vi "isolateNextStringElement.vi"(6 "Final Delimiter":T1, 8 "error in (no error)":errorcluster, 10 "inputString":string, 11 "ILC in":refnum<class "ILC.lvclass">) -> (0 "error out":errorcluster, 1 "remainingString":string, 2 "extractedSegment":string, 3 "ILC out":refnum<class "ILC.lvclass">)   [LabVIEW 2013, in "ILCCommon.lvlib" / "ILC.lvclass"]
uses:
  <userlib>/Common/ILC/ILC/ILC.lvclass
  <userlib>/Common/ILC/ILCModelTypedefs/FinalDelimiter.ctl
  <userlib>/Common/ILC/ILCModelTypedefs/ILCModelTypedefs.lvlib
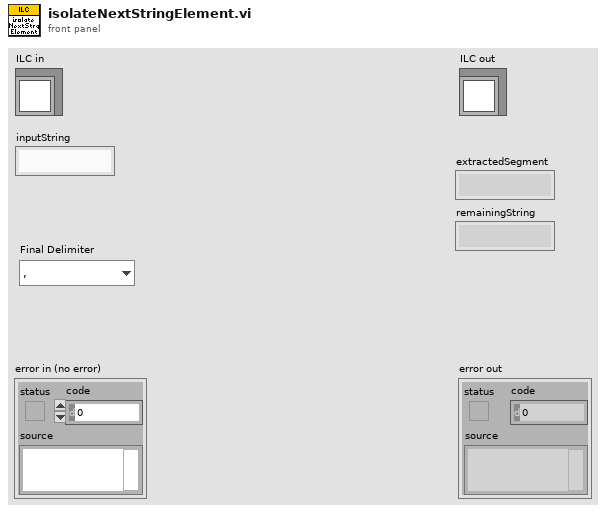
[diagram p1: front panel]
types:
  T1 = typedef "ILCCommon.lvlib/ILCModelTypedefs.lvlib/FinalDelimiter.ctl" = enum16{",", "<CR><LF>"}
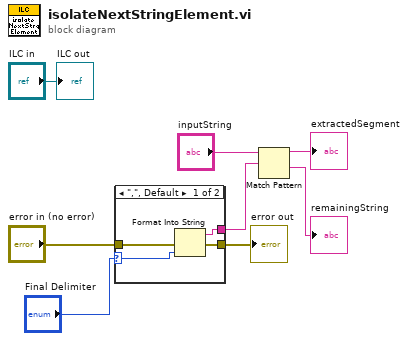
[diagram p0: block diagram]
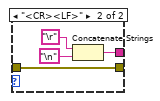
[diagram p2: hidden frame]
diagram:
  n1 = case shown="\",\", Default" "Final Delimiter" {
    selector: "Final Delimiter" -> [w12 _]
    tunnel: [w11 w14] -> w6
    tunnel: "error in (no error)" -> [w10 w13]
    tunnel: [w9 w13] -> w2
    frame ",", Default {
      n2 = Format Into String(error in=w10, w12) -> (resulting string=w11:string, error out=w9:errorcluster)  [unwired: 2 in]
    }
    frame "<CR><LF>" {
      n3 = Concatenate Strings("\r", "\n") -> (w14:string)
    }
  }
  "error out" <- w2
  n4 = Match Pattern(string="inputString", regular expression=w6) -> (before substring=→"extractedSegment":string, after substring=→"remainingString":string)  [unwired: 1 in, 2 out]
  "ILC out" <- "ILC in"
